vi "setFunctionProperties.vi"(2 "error in (no error)":errorcluster, 3 "Function Properties":T1, 4 "AnalogOutput in":refnum<class "AnalogOutput.lvclass">) -> (0 "error out":errorcluster, 1 "AnalogOutput out":refnum<class "AnalogOutput.lvclass">)   [LabVIEW 2011, in "Hardware.lvlib" / "Channels.lvlib" / "AnalogOutput.lvclass"]
uses:
  AnalogOutput.lvclass
  AnalogOutput.lvclass/AnalogOutput.ctl
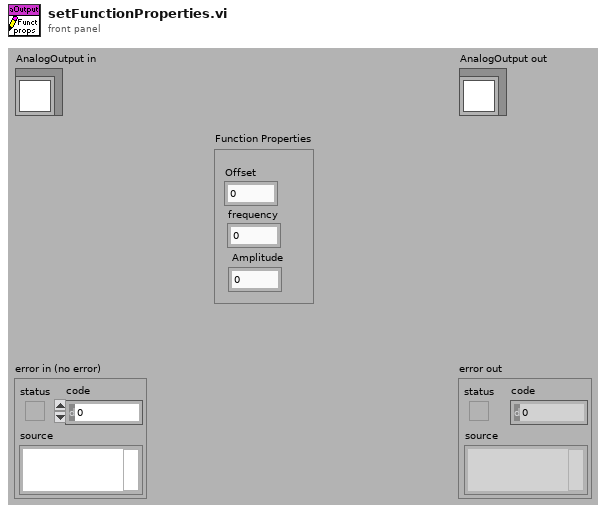
[diagram p1: front panel]
types:
  T1 = cluster{"Offset":dbl, "frequency":dbl, " Amplitude":dbl}
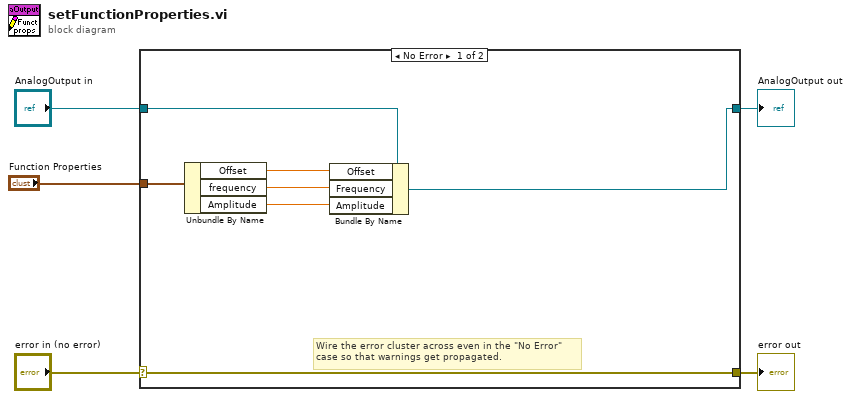
[diagram p0: block diagram]
diagram:
  n1 = case shown="No Error" "error in (no error)" {
    selector: "error in (no error)" -> [w12 w14]
    tunnel: [w12 w14] -> w4
    tunnel: [w10 w13] -> w2
    tunnel: "AnalogOutput in" -> [w11 w13]
    tunnel: "Function Properties" -> [w9 _]
    frame No Error {
      # "Wire the error cluster across even in the \"No Error\"\ncase so that warnings get propagated."
      n2 = Unbundle By Name(w9) -> ("Offset"=w8:dbl, "frequency"=w7:dbl, "Amplitude"=w6:dbl)
      n3 = Bundle By Name(cluster=w11, "Offset"=w8, "Frequency"=w7, "Amplitude"=w6) -> (w10:refnum<class "AnalogOutput.lvclass">)
    }
    frame Error {
    }
  }
  "error out" <- w4
  "AnalogOutput out" <- w2
